vi "Flattened Array to Flattened Elements.vi"(10 "Flattened Array String":string, 11 "Array Type Descriptor":i16[](array[numeric])) -> (2 "Flattened Array Elements":string[](array[string]), 3 "Array Element Type Descriptor":i16[](array[numeric]))   [LabVIEW 2020, in "OpenDescriptor.lvlib"]
uses:
  OpenDescriptor.lvlib
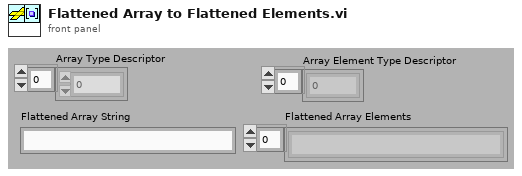
[diagram p1: front panel]
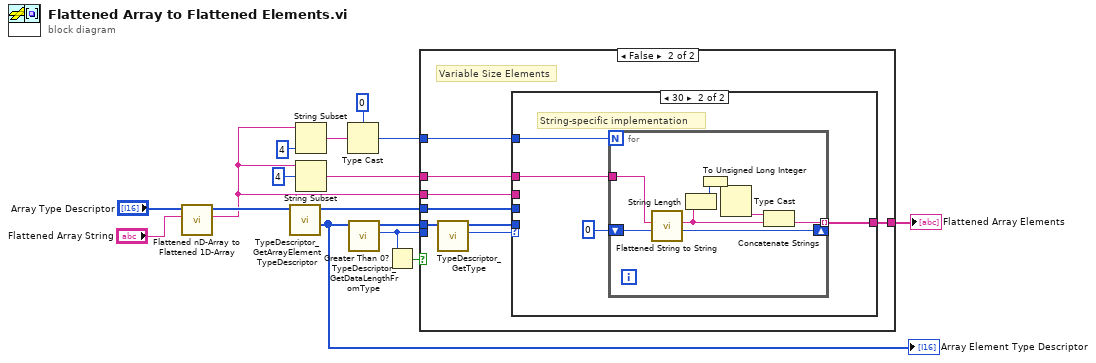
[diagram p0: block diagram]
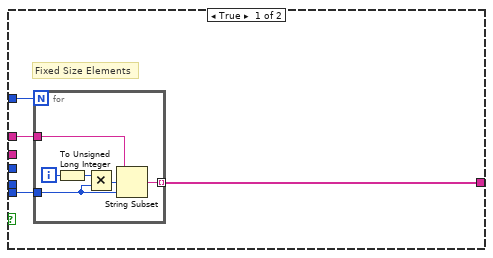
[diagram p2: hidden frame]
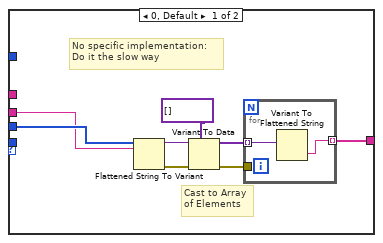
[diagram p3: hidden frame]
diagram:
  n1 = call "Flattened nD-Array to Flattened 1D-Array.vi"("Flattened nD Array"="Flattened Array String", "nD Array Type Descriptor"="Array Type Descriptor") -> ("Flattened 1D Array"=w1:string, "1D Array Type Descriptor"=w2:i16[])  [unwired: 7 in, 1 out]
  n2 = call "TypeDescriptor_GetArrayElementTypeDescriptor.vi"("Array Type Descriptor"=w2) -> ("Element Type Descriptor"=w12:i16[], "Array Type Descriptor dup"=w5:i16[])  [unwired: 9 in]
  "Array Element Type Descriptor" <- w12
  n3 = String Subset(string=w1, length (rest)=4 ("offset (0)")) -> (substring=w10:string)  [unwired: 1 in]
  n4 = String Subset(string=w1, offset (0)=4) -> (substring=w6:string)  [unwired: 1 in]
  n5 = Type Cast(type=0, x=w10) -> (*(type *) &x=w7:i32)
  n6 = call "TypeDescriptor_GetDataLengthFromType.vi"("type descriptor"=w12) -> ("Length"=w14:u32, "type descriptor dup"=w13:i16[])  [unwired: 9 in]
  n7 = Greater Than 0?(x=w14) -> (x > 0?=w15:bool)
  n8 = case shown="False" w15 {
    tunnel: [w20 w34] -> w16
    tunnel: w14 -> [w19 _]
    tunnel: w13 -> [_ w33]
    tunnel: w7 -> [w18 w32]
    tunnel: w6 -> [w17 w31]
    tunnel: w5 -> [_ w28]
    tunnel: w1 -> [_ w27]
    frame True {
      # "Fixed Size Elements"
      n9 = for {
        N: w18 -> [_]
        tunnel: w19 -> [w21]
        tunnel: w17 -> [w25]
        tunnel: [w22] -> w20 mode=indexing
        i -> [w26]
        n10 = To Unsigned Long Integer(number=w26) -> (unsigned 32bit integer=w24:u32)
        n11 = Multiply(x=w24, y=w21) -> (x*y=w23:u32)
        n12 = String Subset(string=w25, offset (0)=w23, length (rest)=w21) -> (substring=w22:string)
      }
    }
    frame False {
      # "Variable Size Elements"
      n13 = call "TypeDescriptor_GetType.vi"("type descriptor"=w33) -> ("Type"=w30:u8, "type descriptor dup"=w29:i16[])  [unwired: 9 in]
      n14 = case shown="30" w30 {
        tunnel: [w38 w48] -> w34
        tunnel: w32 -> [_ w46]
        tunnel: w31 -> [_ w45]
        tunnel: w29 -> [_ _]
        tunnel: w28 -> [w36 _]
        tunnel: w27 -> [w35 _]
        frame 0, Default {
          # "No specific implementation:\nDo it the slow way"
          # "Cast to Array\nof Elements"
          n15 = Flattened String To Variant(6:w35, 7:w36) -> (0:w40:errorcluster, 3:w42:variant)  [unwired: 1 in]
          n16 = Variant To Data(error in=w40, type=variant[] [] ("Elements"), Variant=w42) -> (data=w39:variant[], error out=w37:errorcluster)
          n17 = for {
            tunnel: w39 -> [w44] mode=indexing
            tunnel: [w43] -> w38 mode=indexing
            tunnel: w37 -> [_]
            n18 = Variant To Flattened String(Variant=w44) -> (data string=w43:string)  [unwired: 1 out]
          }
        }
        frame 48 {
          # "String-specific implementation"
          n19 = for {
            N: w46 -> [_]
            tunnel: w45 -> [w52]
            tunnel: [w56] -> w48 mode=indexing
            shift-right: [w49] -> _
            shift-left: u32 0 ("offset (0)") -> [w51]
            n20 = call "Flattened String to String.vi"("Offset"=w51, "Flattened String"=w52) -> ("Offset After String"=w49:u32, "String"=w50:string)  [unwired: 8 in]
            n21 = String Length(string=w50) -> (length=w55:i32)
            n22 = To Unsigned Long Integer(number=w55) -> (unsigned 32bit integer=w54:u32)
            n23 = Type Cast(x=w54) -> (*(type *) &x=w53:string)  [unwired: 1 in]
            n24 = Concatenate Strings(w53, w50) -> (w56:string)
          }
        }
      }
    }
  }
  "Flattened Array Elements" <- w16
